vi "华为UPS2000-G通信.vi"() -> ()   [LabVIEW 2016, in "环境动力监测库.lvlib" / "UPS库.lvlib"]
uses:
  <vilib>/Utility/config.llb/NI_LVConfig.lvlib
panel:
  out "UPS参数":T1 {"开机状态" items=["关机", "开机中", "开机失败", "开机完成"]}
  in  "开机":bool
  out "UPS状态":bool[](array[boolean])
  out "电池状态":T2 {"电池状态" items=["休眠"=2, "浮充"=3, "均充"=4, "放电"=5]}
  in  "open":bool
  in  "close":bool
  out "通信指示":bool
  in  "关机":bool
  in  "状态查询":bool
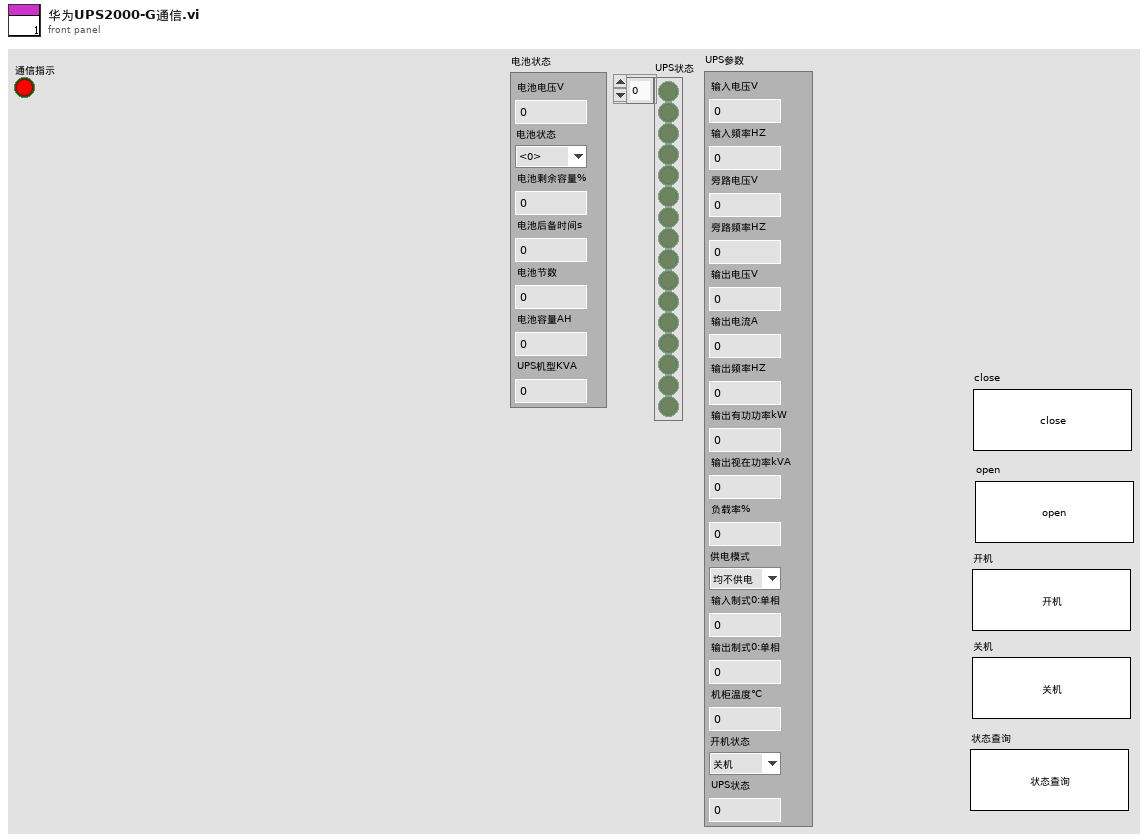
[diagram p1: front panel]
types:
  T1 = cluster{"输入电压V":dbl, "输入频率HZ":dbl, "旁路电压V":dbl, "旁路频率HZ":dbl, "输出电压V":dbl, "输出电流A":dbl, "输出频率HZ":dbl, "输出有功功率kW":dbl, "输出视在功率kVA":dbl, "负载率%":dbl, "供电模式":enum16{"均不供电", "旁路供电", "主路供电", "电池供电", "主路ECO"}, "输入制式0:单相":u16, "输出制式0:单相":u16, "机柜温度℃":dbl, "开机状态":u16, "UPS状态":u8}
  T2 = cluster{"电池电压V":dbl, "电池状态":u16, "电池剩余容量%":u16, "电池后备时间s":u32, "电池节数":u16, "电池容量AH":u16, "UPS机型KVA":u16}
  T3 = typedef "NI_LVConfig.lvlib/Config Data RefNum.ctl" = refnum<k1>
  T4 = cluster{"baud rate (bps)":u32, "stop bits":u16, "parity":u16, "flow control":u16, "timeout":u32, "retries":i32}
  T5 = cluster{"baud rate (9600)":u32, "stop bits (10: 1 bit)":u16, "parity (0:none)":enum16{"None", "Odd", "Even", "Mark", "Space"}, "data bits (8)":u16, "timeout (10sec)":u32}
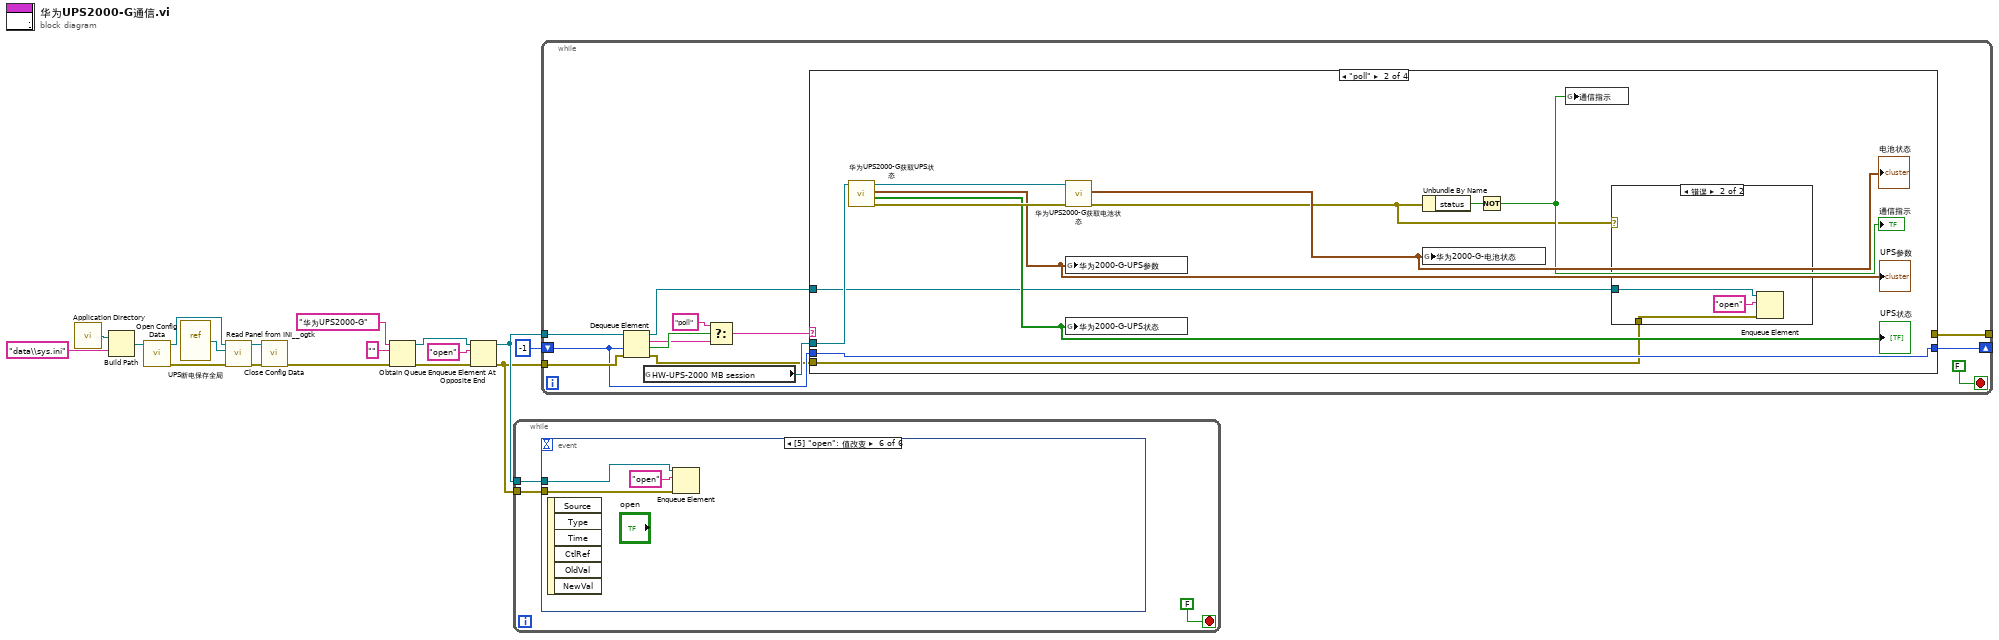
[diagram p0: block diagram]
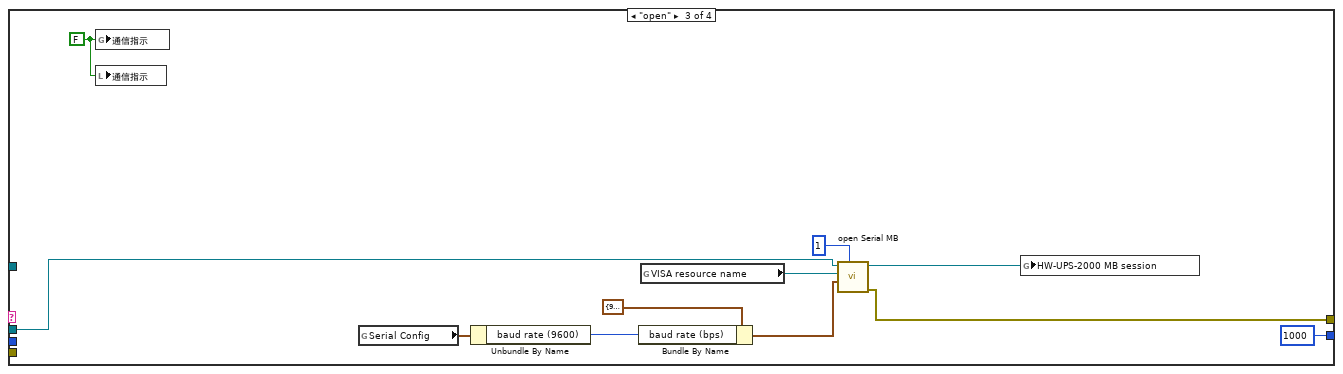
[diagram p4: hidden frame]
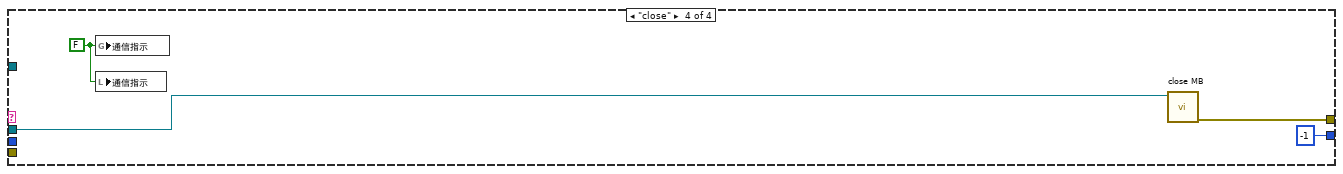
[diagram p5: hidden frame]
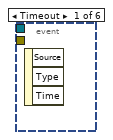
[diagram p6: hidden frame]
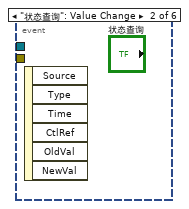
[diagram p7: hidden frame]
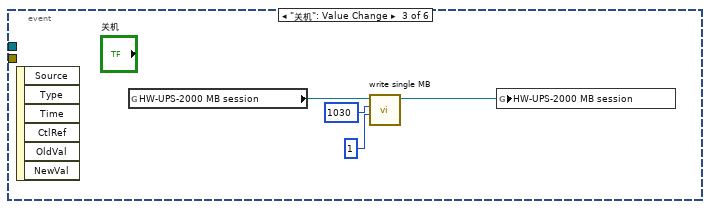
[diagram p8: hidden frame]
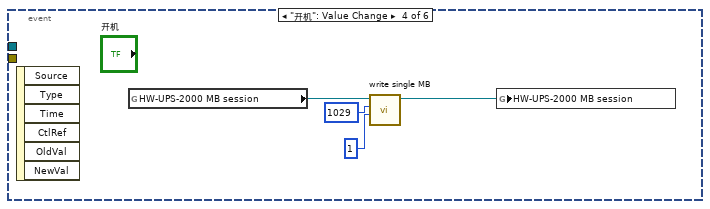
[diagram p9: hidden frame]
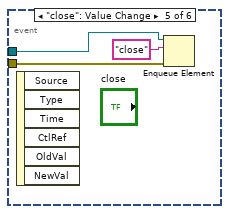
[diagram p10: hidden frame]
diagram:
  n1 = call <vilib>:"Application Directory.vi"() -> ("Application Directory"=w8:path)
  n2 = Build Path(base path=w8, name or relative path="data\\sys.ini" ("名称或相对路径")) -> (appended path=w6:path)
  n3 = call <vilib>:"Open Config Data.vi"("configuration file path"=w6) -> ("error out"=w2:errorcluster, "refnum"=w5:T3)  [unwired: 8 in, 1 out]
  n4 = vi-ref "UPS断电保存全局.vi"() -> (w4:refnum<vi>)
  n5 = call <userlib>:"Read Panel from INI__ogtk.vi"("error in (no error)"=w2, "VI ref"=w4, "refnum"=w5) -> ("error out"=w1:errorcluster, "refnum out"=w3:T3)  [unwired: 7 in]
  n6 = call <vilib>:"Close Config Data.vi"("error in (no error)"=w1, "refnum"=w3) -> ("error out"=w12:errorcluster)  [unwired: 8 in, 1 out]
  n7 = Obtain Queue(name (unnamed)="华为UPS2000-G" ("名称（未命名）"), element data type="", error in (no error)=w12) -> (queue out=w14:refnum<queue>, error out=w13:errorcluster)  [unwired: 2 in, 1 out]
  n8 = Enqueue Element At Opposite End(queue=w14, element="open" ("元素"), error in (no error)=w13) -> (queue out=w10:refnum<queue>, error out=w9:errorcluster)  [unwired: 1 in, 1 out]
  n9 = while {
    tunnel: w10 -> [w19]
    tunnel: w9 -> [w18]
    stop <- FALSE stop-if-true
    n10 = event shown="[5] \"open\": 值改变" {
      selector: _ -> [_ _ _ _ _ _]
      dyn-events: _ -> [_ _ _ _ _ _]
      timeout: _ -> [_ _ _ _ _ _]
      tunnel: w19 -> [_ _ _ _ w30 w33]
      tunnel: w18 -> [_ _ _ _ w29 w32]
      event Timeout {
        n11 = event-data() -> ()  [unwired: 1 in, 3 out]
      }
      event "状态查询": Value Change {
        n12 = event-data() -> ()  [unwired: 1 in, 6 out]
      }
      event "关机": Value Change {
        n13 = event-data() -> ()  [unwired: 1 in, 6 out]
        n14 = global read "UPS断电保存全局.vi" "HW-UPS-2000 MB session"() -> (w23:refnum<class "MB_Master.lvclass">)
        n15 = call "write single MB.vi"("value"=u16 1, "address"=u16 1030, "MB session in"=w23) -> ("MB session out"=w24:refnum<class "MB_Master.lvclass">)  [unwired: 7 in, 1 out]
        n16 = global write "UPS断电保存全局.vi" "HW-UPS-2000 MB session"(w24) -> ()
      }
      event "开机": Value Change {
        n17 = event-data() -> ()  [unwired: 1 in, 6 out]
        n18 = global read "UPS断电保存全局.vi" "HW-UPS-2000 MB session"() -> (w27:refnum<class "MB_Master.lvclass">)
        n19 = call "write single MB.vi"("value"=u16 1, "address"=u16 1029, "MB session in"=w27) -> ("MB session out"=w28:refnum<class "MB_Master.lvclass">)  [unwired: 7 in, 1 out]
        n20 = global write "UPS断电保存全局.vi" "HW-UPS-2000 MB session"(w28) -> ()
      }
      event "close": Value Change {
        n21 = event-data() -> ()  [unwired: 1 in, 6 out]
        n22 = Enqueue Element(queue=w30, element="close" ("元素"), error in (no error)=w29) -> ()  [unwired: 1 in, 3 out]
      }
      event "open": Value Change {
        n23 = event-data() -> ()  [unwired: 1 in, 6 out]
        n24 = Enqueue Element(queue=w33, element="open" ("元素"), error in (no error)=w32) -> ()  [unwired: 1 in, 3 out]
      }
    }
  }
  n25 = while {
    tunnel: w10 -> [w44]
    tunnel: w9 -> [w43]
    shift-right: [w40] -> _
    shift-left: -1 ("超时毫秒(-1)") -> [w41]
    tunnel: [w38] -> _
    stop <- FALSE stop-if-true
    n26 = Dequeue Element(queue=w44, timeout in ms (-1)=w41, error in (no error)=w43) -> (queue out=w36:refnum<queue>, element=w45:string, timed out?=w47:bool, error out=w35:errorcluster)
    n27 = global read "UPS断电保存全局.vi" "HW-UPS-2000 MB session"() -> (w39:refnum<class "MB_Master.lvclass">)
    n28 = Select(t="poll" ("元素"), s=w47, f=w45) -> (s? t:f=w42:string)
    n29 = case shown="\"poll\"" w42 {
      tunnel: w41 -> [w48 w60 _ _]
      tunnel: [w48 w60 1000 ("超时毫秒(-1)") -1 ("超时毫秒(-1)")] -> w40
      tunnel: w39 -> [_ w59 w67 w77]
      tunnel: [_ _ w65 w75] -> w38
      tunnel: w36 -> [_ w50 _ _]
      tunnel: w35 -> [_ w49 _ _]
      frame Default {
      }
      frame "poll" {
        n30 = call "华为UPS2000-G获取UPS状态.vi"("MB session in"=w59) -> ("error out"=w57:errorcluster, "UPS状态"=w54:bool[], "UPS参数"=w55:T1, "MB session out"=w58:refnum<class "MB_Master.lvclass">)  [unwired: 7 in]
        "UPS状态" <- w54
        "UPS参数" <- w55
        n31 = call "华为UPS2000-G获取电池状态.vi"("error in (no error)"=w57, "MB session in"=w58) -> ("error out"=w51:errorcluster, "电池状态"=w53:T2)  [unwired: 7 in, 1 out]
        "电池状态" <- w53
        n32 = global write "UPS内部交互全局.vi" "华为2000-G-UPS参数"(w55) -> ()
        n33 = global write "UPS内部交互全局.vi" "华为2000-G-UPS状态"(w54) -> ()
        n34 = Unbundle By Name(w51) -> ("status"=w56:bool)
        n35 = global write "UPS内部交互全局.vi" "华为2000-G-电池状态"(w53) -> ()
        n36 = Not(x=w56) -> (.not. x?=w52:bool)
        "通信指示" <- w52
        n37 = global write "UPS内部交互全局.vi" "通信指示"(w52) -> ()
        n38 = case shown="错误" w51 {
          tunnel: w50 -> [_ w62]
          tunnel: w49 -> [_ w61]
          frame No Error {
          }
          frame Error {
            n39 = Enqueue Element(queue=w62, element="open" ("元素"), error in (no error)=w61) -> ()  [unwired: 1 in, 3 out]
          }
        }
      }
      frame "open" {
        w64 = FALSE ("通讯状态 2")
        n40 = global write "UPS内部交互全局.vi" "通信指示"(w64) -> ()
        n41 = local write "通信指示"(w64) -> ()
        n42 = global read "UPS断电保存全局.vi" "Serial Config"() -> (w71:T5)
        n43 = Unbundle By Name(w71) -> ("baud rate (9600)"=w70:u32)
        n44 = Bundle By Name(cluster=T4 {"baud rate (bps)"=9600, "stop bits"=10, "parity"=0, "flow control"=0, "timeout"=1000, "retries"=1} ("Serial Config"), "baud rate (bps)"=w70) -> (w69:T4)
        n45 = global read "UPS断电保存全局.vi" "VISA resource name"() -> (w73:refnum<visa-resource-name>)
        n46 = call "open Serial MB.vi"("Slave ID"=u8 1, "Serial Config"=w69, "VISA Resource"=w73, "MB session in"=w67) -> ("error out"=w65:errorcluster, "MB session out"=w68:refnum<class "MB_Master.lvclass">)  [unwired: 6 in]
        n47 = global write "UPS断电保存全局.vi" "HW-UPS-2000 MB session"(w68) -> ()
      }
      frame "close" {
        w78 = FALSE ("通讯状态 2")
        n48 = global write "UPS内部交互全局.vi" "通信指示"(w78) -> ()
        n49 = local write "通信指示"(w78) -> ()
        n50 = call "close MB.vi"("MB session in"=w77) -> ("error out"=w75:errorcluster)  [unwired: 10 in]
      }
    }
  }
